vi "例6.4 利用波形文件io保存波形.vi"() -> ()   [LabVIEW 2017]
uses:
  <vilib>/Waveform/WDTFileIO.llb/ Write Waveform to File.vi
  <vilib>/measure/NI_MABase.lvlib
panel:
  out "first waveform in record":waveform(dbl) caption="记录中第一波形"
  out "波形图":waveform(dbl)(graph)
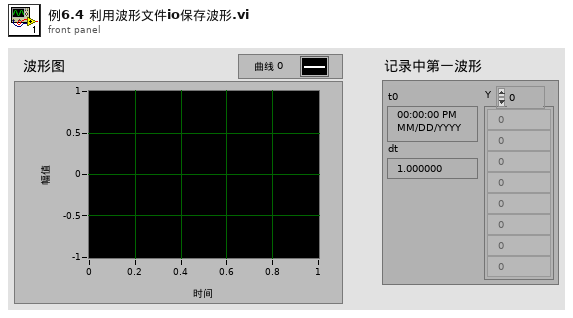
[diagram p1: front panel]
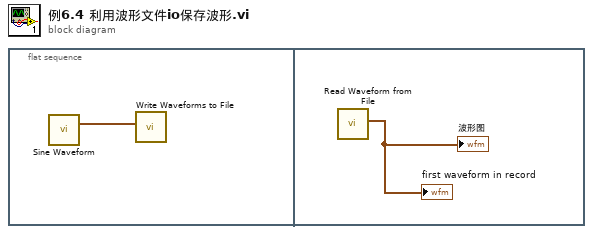
[diagram p0: block diagram]
diagram:
  n1 = flat-sequence {
    frame #0 {
      n2 = call <vilib>:"Sine Waveform.vi"() -> ("signal out"=w1:waveform(dbl))  [unwired: 10 in, 1 out]
      n3 = call-poly <vilib>:"Write Waveforms to File.vi"("waveform"=w1) -> ()  [unwired: 9 in, 2 out]
    }
    frame #1 {
      n4 = call <vilib>:"Read Waveform from File.vi"() -> ("first waveform in record"=→"波形图" →"first waveform in record":waveform(dbl))  [unwired: 6 in, 3 out]
    }
  }
